vi "Update Value.vi"(6 "Time":dbl, 8 "error in (no error)":errorcluster, 11 "LoggingControl in":refnum<class "GroupLoggingControl.lvclass">) -> (0 "error out":errorcluster, 1 "Update":bool, 2 "Value":variant, 3 "LoggingControl out":refnum<class "GroupLoggingControl.lvclass">)   [LabVIEW 2020, in "VolatusGUIElements.lvlib" / "GroupLoggingControl.lvclass"]
uses:
  GroupLoggingControl.lvclass
  GroupLoggingControl.lvclass/GroupLoggingControl.ctl
  lv-vecto/Vecto/Channel STR/Channel STR.lvclass
  VolatusData/Logging State.ctl
  VolatusData/VolatusData.lvlib
  <vilib>/Utility/miscctls.llb/LVMapReplaceAction.ctl
  lv-vecto/Vecto/Channel DBL/Channel DBL.lvclass
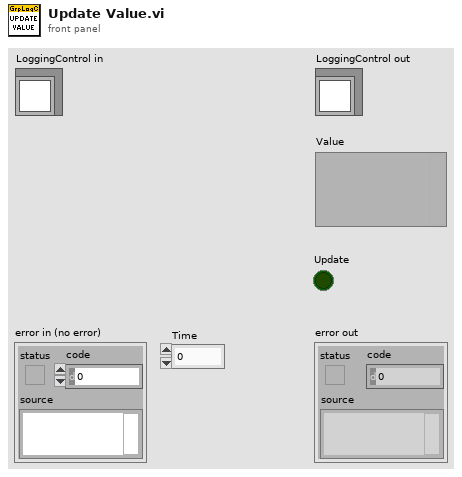
[diagram p1: front panel]
types:
  T1 = cluster{"Group":string, "Group Color":u32, "Button":bool}[]
  T2 = typedef "LVMapReplaceAction.ctl" = enum32{"Modify Entry only if found", "Add or Modify Entry", "Delete Entry"}
  T3 = typedef "VolatusData.lvlib/Logging State.ctl" = enum16{"Idle", "Starting", "Logging", "Stopping"}
  T4 = cluster{"Series":string, "Timestamp":string, "Targets":cluster{"Node":string, "Node Color":u32, "Groups":cluster{"Group":string, "Group Color":u32, "Button":bool}[]}[], "Groups":cluster{"Group":string, "Group Color":u32, "Button":bool}[]}
  T5 = typedef "VolatusGUIElements.lvlib/GroupLoggingControl.lvclass/Target Info.ctl" = cluster{"Node":string, "Node Color":u32, "Groups":T6[]}
  T6 = typedef "VolatusGUIElements.lvlib/GroupLoggingControl.lvclass/Log Group.ctl" = cluster{"Status":T7, "Command Info":T8, "Logging":bool, "State":string}
  T7 = typedef "VolatusGUIElements.lvlib/GroupLoggingControl.lvclass/Log Group Status.ctl" = cluster{"Group":string, "Group Color":u32, "Button":bool}
  T8 = typedef "VolatusGUIElements.lvlib/GroupLoggingControl.lvclass/Command Info.ctl" = cluster{"Commanding":bool, "Cmd Time":dbl, "Group ID":string}
  T9 = typedef "VolatusGUIElements.lvlib/GroupLoggingControl.lvclass/Log State.ctl" = cluster{"Series":string, "Timestamp":string, "Requested":bool}
  T10 = cluster{"Group":string, "Group Color":u32, "Button":bool}
  T11 = cluster{"Node":string, u32, cluster{"Group":string, "Group Color":u32, "Button":bool}[]}
  T12 = cluster{string, string, cluster{"Node":string, u32, cluster{"Group":string, "Group Color":u32, "Button":bool}[]}[], "Groups":cluster{"Group":string, "Group Color":u32, "Button":bool}[]}
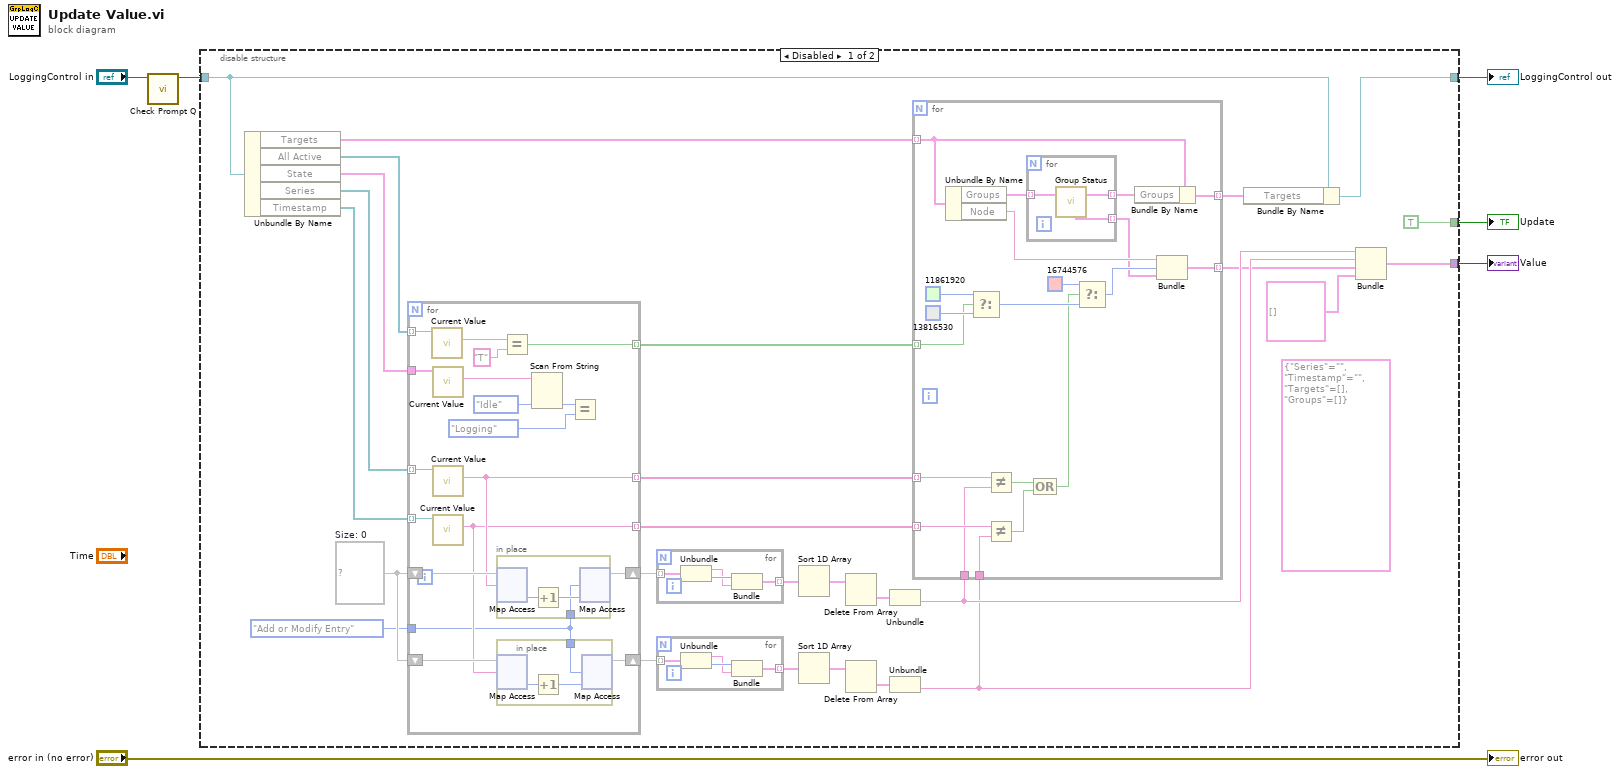
[diagram p0: block diagram]
diagram:
  n1 = call "Check Prompt Q.vi"("LoggingControl in"="LoggingControl in") -> ("LoggingControl out"=w2:refnum<class "GroupLoggingControl.lvclass">)  [unwired: 9 in, 1 out]
  n2 = disable-structure shown="Disabled" {
    disable-tunnel: [TRUE ("Update") _] -> w4
    disable-tunnel: [w32 _] -> w3
    disable-tunnel: w2 -> [w12 w89]
    disable-tunnel: [w8 w89] -> w1
    frame Disabled {
      (unwired) T4 {"Series"="", "Timestamp"="", "Targets"=[], "Groups"=[]} ("Group Logging Control")
      w23 = map{string, i32} {}  # Size: 0
      n3 = Unbundle By Name(w12) -> ("Targets"=w24:T5[], "All Active"=w31:refnum<class "Channel DBL.lvclass">[], "State"=w30:T9, "Series"=w29:refnum<class "Channel STR.lvclass">[], "Timestamp"=w28:refnum<class "Channel STR.lvclass">[])
      n4 = for {
        tunnel: w31 -> [w48] mode=indexing
        tunnel: w30 -> [w49]
        tunnel: w29 -> [w45] mode=indexing
        tunnel: w28 -> [w44] mode=indexing
        tunnel: [w40] -> w26 mode=indexing
        tunnel: [w36] -> w25 mode=indexing
        tunnel: [w43] -> w27 mode=indexing
        shift-right: [w39] -> w22
        shift-left: w23 -> [w41]
        shift-right: [w38] -> w21
        shift-left: w23 -> [w37]
        tunnel: LVMapReplaceAction."Add or Modify Entry" ("action") -> [w34]
        n5 = call "Current Value.vi"("StringChannel in"=w48) -> ("String"=w47:string)  [unwired: 7 in, 3 out]
        n6 = call "Current Value.vi"("StringChannel in"=w49) -> ("String"=w42:string)  [unwired: 7 in, 3 out]
        n7 = call "Current Value.vi"("StringChannel in"=w45) -> ("String"=w40:string)  [unwired: 7 in, 3 out]
        n8 = call "Current Value.vi"("StringChannel in"=w44) -> ("String"=w36:string)  [unwired: 7 in, 3 out]
        n9 = in-place {
          in-place-border: w34 -> [w52]
          n10 = in-place-map #1(w41, w40) -> (w54:i32)  [unwired: 1 in, 1 out]
          n11 = Increment(x=w54) -> (x+1=w53:i32)
          n12 = in-place-map #1(w53, w52) -> (w39:map{string, i32})  [unwired: 2 out]
        }
        n13 = in-place {
          in-place-border: w34 -> [w55]
          n14 = in-place-map #2(w37, w36) -> (w57:i32)  [unwired: 1 in, 1 out]
          n15 = Increment(x=w57) -> (x+1=w56:i32)
          n16 = in-place-map #2(w56, w55) -> (w38:map{string, i32})  [unwired: 2 out]
        }
        n17 = Equal?(x=w47, y="T") -> (x = y?=w43:bool)
        n18 = Scan From String(input string=w42, default 1=Logging_State."Idle" ("Logging State")) -> (output 1=w51:T3)  [unwired: 3 in, 3 out]
        n19 = Equal?(x=w51, y=Logging_State."Logging" ("Logging State")) -> ()  [unwired: 1 out]
      }
      n20 = for {
        tunnel: w22 -> [w84] mode=indexing
        tunnel: [w81] -> w19 mode=indexing
        n21 = Unbundle(w84) -> (w82:string, w83:i32)
        n22 = Bundle(w83, w82) -> (w81:cluster{i32, string})  [unwired: 1 in]
      }
      n23 = for {
        tunnel: w21 -> [w88] mode=indexing
        tunnel: [w85] -> w20 mode=indexing
        n24 = Unbundle(w88) -> (w86:string, w87:i32)
        n25 = Bundle(w87, w86) -> (w85:cluster{i32, string})  [unwired: 1 in]
      }
      n26 = Sort 1D Array(array=w19) -> (sorted array=w17:cluster{i32, string}[])
      n27 = Sort 1D Array(array=w20) -> (sorted array=w18:cluster{i32, string}[])
      n28 = Delete From Array(array=w17) -> (deleted portion=w16:cluster{i32, string})  [unwired: 2 in, 1 out]
      n29 = Delete From Array(array=w18) -> (deleted portion=w15:cluster{i32, string})  [unwired: 2 in, 1 out]
      n30 = Unbundle(w16) -> (w14:string)  [unwired: 1 out]
      n31 = Unbundle(w15) -> (w13:string)  [unwired: 1 out]
      n32 = for {
        tunnel: w27 -> [w75] mode=indexing
        tunnel: w26 -> [w72] mode=indexing
        tunnel: w25 -> [w71] mode=indexing
        tunnel: w24 -> [w60] mode=indexing
        tunnel: w14 -> [w70]
        tunnel: w13 -> [w69]
        tunnel: [w64] -> w10 mode=indexing
        tunnel: [w58] -> w7 mode=indexing
        n33 = Unbundle By Name(w60) -> ("Groups"=w62:T6[], "Node"=w63:string)
        n34 = Select(t=u32 11861920, s=w75, f=u32 13816530) -> (s? t:f=w74:u32)
        n35 = Not Equal?(x=w72, y=w70) -> (x != y?=w68:bool)
        n36 = Not Equal?(x=w71, y=w69) -> (x != y?=w67:bool)
        n37 = for {
          tunnel: w62 -> [w80] mode=indexing
          tunnel: [w79] -> w61 mode=indexing
          tunnel: [w78] -> w59 mode=indexing
          n38 = call "Group Status.vi"("Log Group"=w80) -> ("Group Status"=w79:T10, "Group"=w78:T6)  [unwired: 5 in]
        }
        n39 = Compound Arithmetic op=OR(w68, w67) -> (w66:bool)
        n40 = Select(t=u32 16744576, s=w66, f=w74) -> (s? t:f=w65:u32)
        n41 = Bundle By Name(cluster=w60, "Groups"=w59) -> (w58:T5)
        n42 = Bundle("Node"=w63, w65, w61) -> (w64:T11)  [unwired: 1 in]
      }
      n43 = Bundle By Name(cluster=w12, "Targets"=w7) -> (w8:refnum<class "GroupLoggingControl.lvclass">)
      n44 = Bundle(w14, w13, w10, "Groups"=T1 []) -> (w32:T12)  [unwired: 1 in]
    }
    frame Enabled {
    }
  }
  "LoggingControl out" <- w1
  "Value" <- w3
  "Update" <- w4
  "error out" <- "error in (no error)"
